vi "Initialize GUI (SubVI).vi"(0 "References IN":T1, 9 "Initialize Command":bool) -> (4 "References OUT":T1)   [LabVIEW 2010]
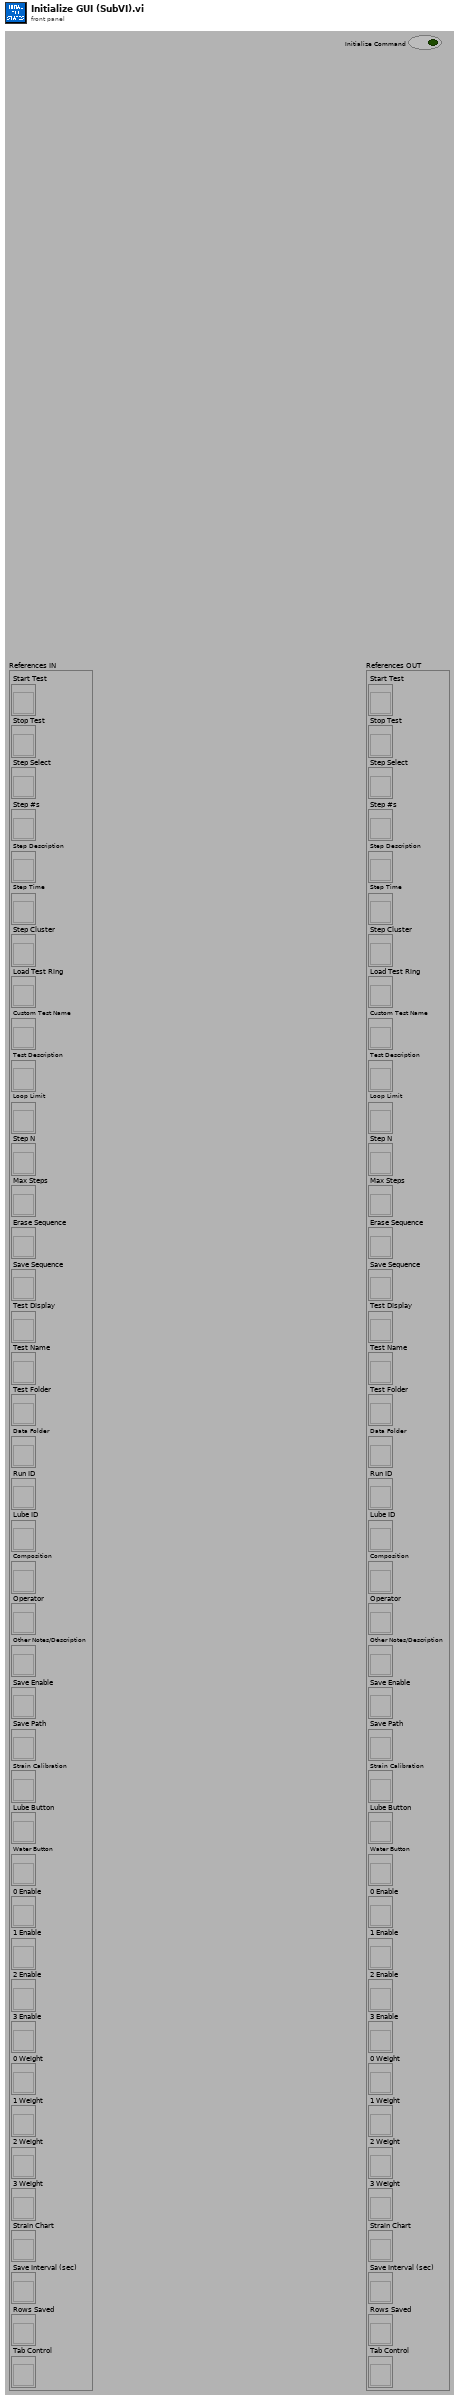
[diagram p1: front panel]
types:
  T1 = cluster{"Start Test":refnum<vi>, "Stop Test":refnum<vi>, "Step Select":refnum<vi>, "Step #s":refnum<vi>, "Step Description":refnum<vi>, "Step Time":refnum<vi>, "Step Cluster":refnum<vi>, "Load Test Ring":refnum<vi>, "Custom Test Name":refnum<vi>, "Test Description":refnum<vi>, "Loop Limit":refnum<vi>, "Step N":refnum<vi>, "Max Steps":refnum<vi>, "Erase Sequence":refnum<vi>, "Save Sequence":refnum<vi>, "Test Display":refnum<vi>, "Test Name":refnum<vi>, "Test Folder":refnum<vi>, "Data Folder":refnum<vi>, "Run ID":refnum<vi>, "Lube ID":refnum<vi>, "Composition":refnum<vi>, "Operator":refnum<vi>, "Other Notes/Description":refnum<vi>, "Save Enable":refnum<vi>, "Save Path":refnum<vi>, "Strain Calibration":refnum<vi>, "Lube Button":refnum<vi>, "Water Button":refnum<vi>, "0 Enable":refnum<vi>, "1 Enable":refnum<vi>, "2 Enable":refnum<vi>, "3 Enable":refnum<vi>, "0 Weight":refnum<vi>, "1 Weight":refnum<vi>, "2 Weight":refnum<vi>, "3 Weight":refnum<vi>, "Strain Chart":refnum<vi>, "Save Interval (sec)":refnum<vi>, "Rows Saved":refnum<vi>, "Tab Control":refnum<vi>}
  T2 = enum8{"Enabled", "Disabled", "Disabled and Grayed Out"}
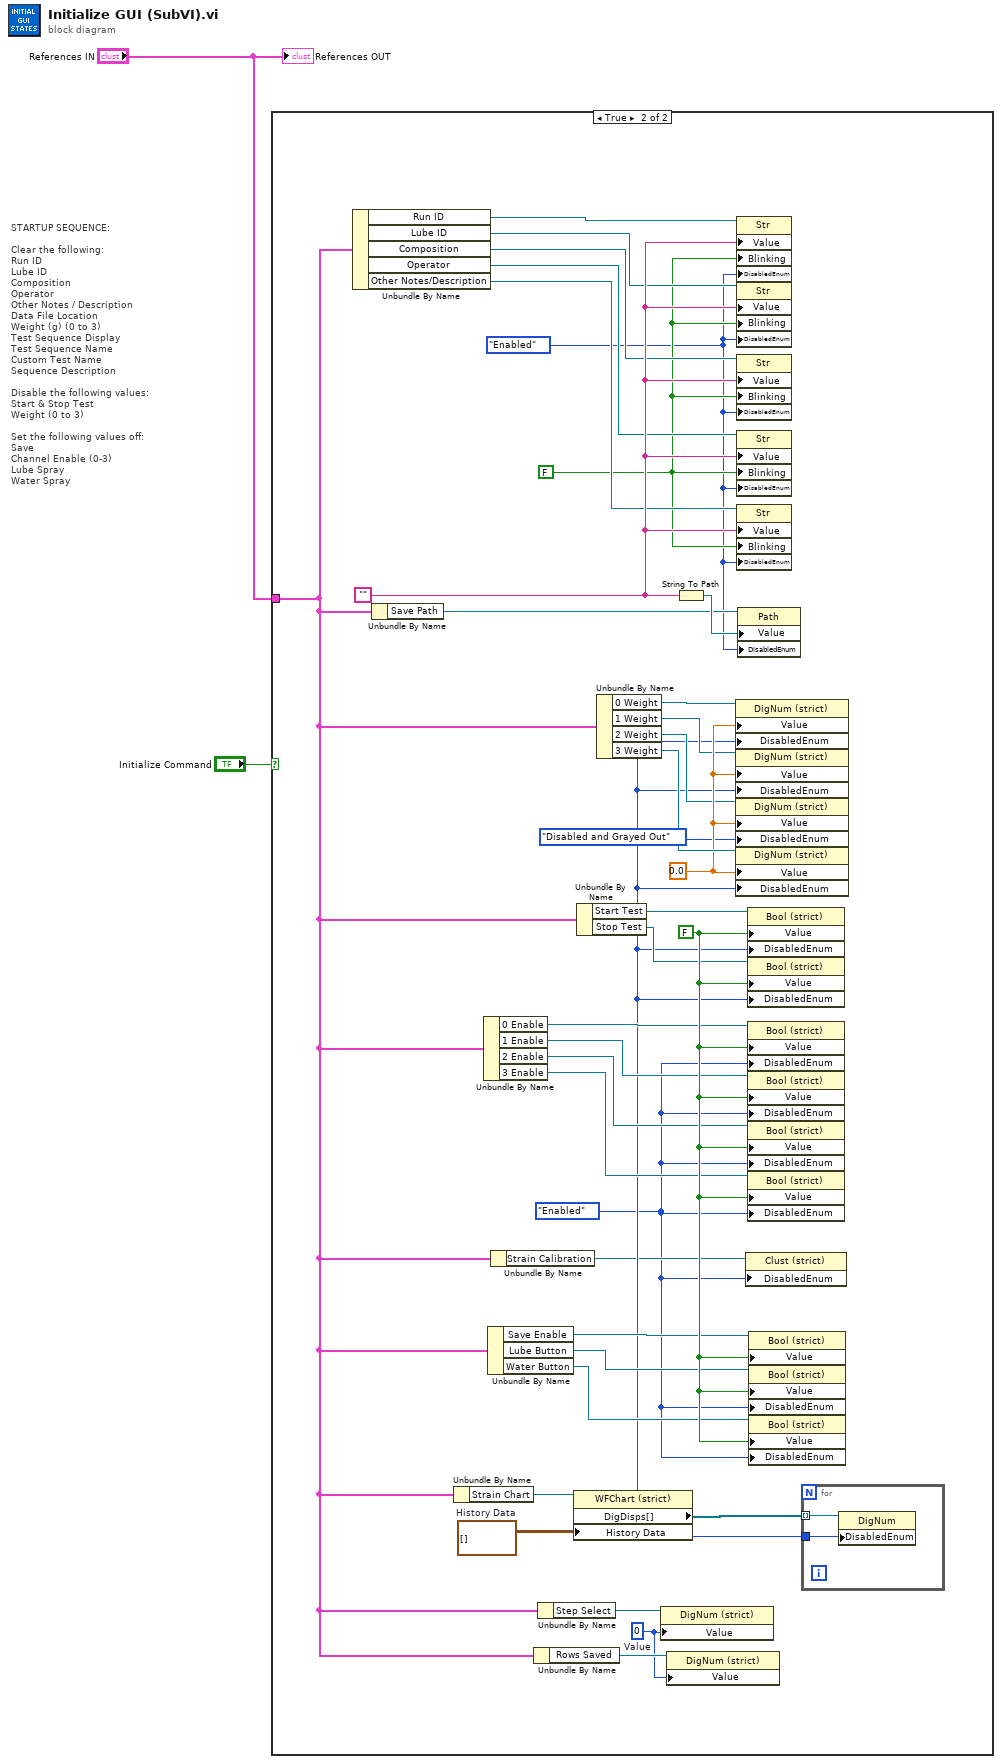
[diagram p0: block diagram]
diagram:
  # "STARTUP SEQUENCE:\n\nClear the following:\nRun ID\nLube ID\nComposition\nOperator\nOther Notes / Description\nData File Location\nWeight (g) (0 to 3)\nTest Sequence Display\nTest Sequence Name\nCustom Test Name\nSequence Description\n\nDisable the following values:\nStart & Stop Test\nWeight (0 to 3)\n\nSet the following values off:\nSave\nChannel Enable (0-3)\nLube Spray\nWater Spray"
  n1 = case shown="True" "Initialize Command" {
    tunnel: "References IN" -> [_ w6]
    frame False {
    }
    frame True {
      w4 = waveform(dbl)[][] []  # History Data
      w3 = T2."Enabled" ("Disabled")
      w8 = T2."Enabled" ("Disabled")
      w10 = FALSE
      w5 = 0  # Value
      w36 = FALSE ("Value")
      w13 = T2."Disabled and Grayed Out" ("Disabled")
      w25 = 0.0 ("Value")
      w37 = "" ("Value")
      n2 = Unbundle By Name(w6) -> ("Run ID"=w17:refnum<vi>, "Lube ID"=w18:refnum<vi>, "Composition"=w19:refnum<vi>, "Operator"=w20:refnum<vi>, "Other Notes/Description"=w21:refnum<vi>)
      n3 = Unbundle By Name(w6) -> ("Save Path"=w11:refnum<vi>)
      n4 = Unbundle By Name(w6) -> ("Strain Chart"=w16:refnum<vi>)
      n5 = Unbundle By Name(w6) -> ("0 Enable"=w29:refnum<vi>, "1 Enable"=w30:refnum<vi>, "2 Enable"=w31:refnum<vi>, "3 Enable"=w32:refnum<vi>)
      n6 = Unbundle By Name(w6) -> ("Save Enable"=w33:refnum<vi>, "Lube Button"=w34:refnum<vi>, "Water Button"=w35:refnum<vi>)
      n7 = Unbundle By Name(w6) -> ("Strain Calibration"=w9:refnum<vi>)
      n8 = Unbundle By Name(w6) -> ("Rows Saved"=w7:refnum<vi>)
      n9 = Unbundle By Name(w6) -> ("Step Select"=w14:refnum<vi>)
      n10 = property class="WFChart (strict)"(reference=w16, "History Data"=w4) -> ("DigDisps[]"=w15:refnum<vi>[])  [unwired: 1 in, 2 out]
      n11 = Unbundle By Name(w6) -> ("Start Test"=w27:refnum<vi>, "Stop Test"=w28:refnum<vi>)
      n12 = Unbundle By Name(w6) -> ("0 Weight"=w22:refnum<vi>, "1 Weight"=w23:refnum<vi>, "2 Weight"=w24:refnum<vi>, "3 Weight"=w26:refnum<vi>)
      n13 = property class="DigNum (strict)"(reference=w14, "Value"=w5) -> ()  [unwired: 1 in, 2 out]
      n14 = property class="DigNum (strict)"(reference=w7, "Value"=w5) -> ()  [unwired: 1 in, 2 out]
      n15 = String To Path(string=w37) -> (path=w12:path)
      n16 = property class="DigNum (strict)"(reference=w22, "Value"=w25, "DisabledEnum"=w13) -> ()  [unwired: 1 in, 2 out]
      n17 = property class="DigNum (strict)"(reference=w23, "Value"=w25, "DisabledEnum"=w13) -> ()  [unwired: 1 in, 2 out]
      n18 = property class="DigNum (strict)"(reference=w24, "Value"=w25, "DisabledEnum"=w13) -> ()  [unwired: 1 in, 2 out]
      n19 = property class="DigNum (strict)"(reference=w26, "Value"=w25, "DisabledEnum"=w13) -> ()  [unwired: 1 in, 2 out]
      n20 = property class="Str"(reference=w17, "Value"=w37, "Blinking"=w10, "DisabledEnum"=w8) -> ()  [unwired: 1 in, 2 out]
      n21 = property class="Str"(reference=w18, "Value"=w37, "Blinking"=w10, "DisabledEnum"=w8) -> ()  [unwired: 1 in, 2 out]
      n22 = property class="Str"(reference=w19, "Value"=w37, "Blinking"=w10, "DisabledEnum"=w8) -> ()  [unwired: 1 in, 2 out]
      n23 = property class="Str"(reference=w20, "Value"=w37, "Blinking"=w10, "DisabledEnum"=w8) -> ()  [unwired: 1 in, 2 out]
      n24 = property class="Str"(reference=w21, "Value"=w37, "Blinking"=w10, "DisabledEnum"=w8) -> ()  [unwired: 1 in, 2 out]
      n25 = property class="Path"(reference=w11, "Value"=w12, "DisabledEnum"=w8) -> ()  [unwired: 1 in, 2 out]
      n26 = property class="Clust (strict)"(reference=w9, "DisabledEnum"=w3) -> ()  [unwired: 1 in, 2 out]
      n27 = property class="Bool (strict)"(reference=w27, "Value"=w36, "DisabledEnum"=w13) -> ()  [unwired: 1 in, 2 out]
      n28 = property class="Bool (strict)"(reference=w28, "Value"=w36, "DisabledEnum"=w13) -> ()  [unwired: 1 in, 2 out]
      n29 = property class="Bool (strict)"(reference=w29, "Value"=w36, "DisabledEnum"=w3) -> ()  [unwired: 1 in, 2 out]
      n30 = property class="Bool (strict)"(reference=w30, "Value"=w36, "DisabledEnum"=w3) -> ()  [unwired: 1 in, 2 out]
      n31 = property class="Bool (strict)"(reference=w31, "Value"=w36, "DisabledEnum"=w3) -> ()  [unwired: 1 in, 2 out]
      n32 = property class="Bool (strict)"(reference=w32, "Value"=w36, "DisabledEnum"=w3) -> ()  [unwired: 1 in, 2 out]
      n33 = property class="Bool (strict)"(reference=w33, "Value"=w36) -> ()  [unwired: 1 in, 2 out]
      n34 = property class="Bool (strict)"(reference=w34, "Value"=w36, "DisabledEnum"=w3) -> ()  [unwired: 1 in, 2 out]
      n35 = property class="Bool (strict)"(reference=w35, "Value"=w36, "DisabledEnum"=w3) -> ()  [unwired: 1 in, 2 out]
      n36 = for {
        tunnel: w15 -> [w39] mode=indexing
        tunnel: w13 -> [w38]
        n37 = property class="DigNum"(reference=w39, "DisabledEnum"=w38) -> ()  [unwired: 1 in, 2 out]
      }
    }
  }
  "References OUT" <- "References IN"
